vi "ReadBuffer.vi"(8 "error in (no error)":errorcluster, 11 "Arduino in":refnum<class "Arduino.lvclass">) -> (0 "error out":errorcluster, 2 "New Data Found":bool, 3 "Arduino out":refnum<class "Arduino.lvclass">)   [LabVIEW 2014, in "Arduino.lvclass"]
uses:
  Arduino.lvclass
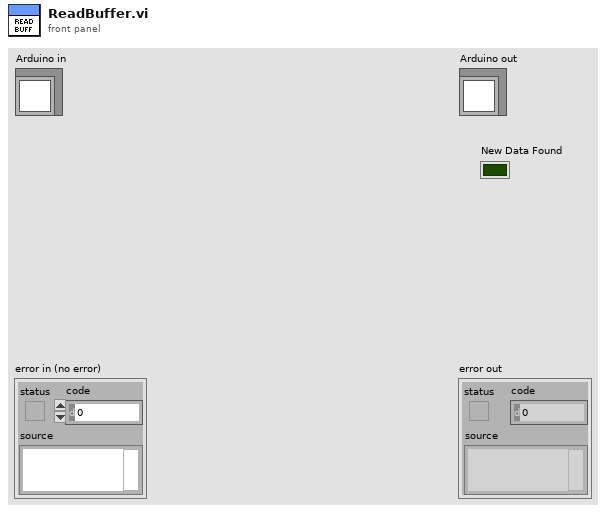
[diagram p1: front panel]
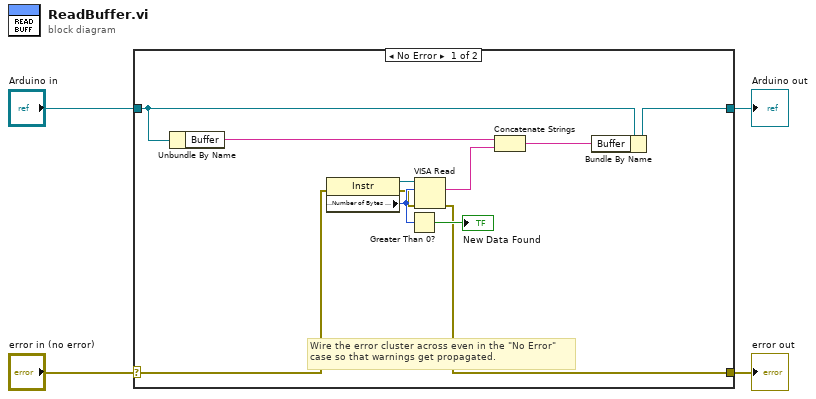
[diagram p0: block diagram]
diagram:
  n1 = case shown="No Error" "error in (no error)" {
    selector: "error in (no error)" -> [w10 w17]
    tunnel: [w11 w17] -> w3
    tunnel: [w5 w16] -> w1
    tunnel: "Arduino in" -> [w6 w16]
    frame No Error {
      # "Wire the error cluster across even in the \"No Error\"\ncase so that warnings get propagated."
      n2 = Unbundle By Name(w6) -> ("Buffer"=w8:string)
      n3 = property class="Instr"(error in=w10) -> (reference out=w15:refnum<visa-resource-name>, error out=w12:errorcluster, "Serial Settings:Number of Bytes at Serial Port"=w14:u32)  [unwired: 1 in]
      n4 = Greater Than 0?(x=w14) -> (x > 0?=→"New Data Found":bool)
      n5 = VISA Read(VISA resource name=w15, byte count=w14, error in (no error)=w12) -> (read buffer=w9:string, error out=w11:errorcluster)  [unwired: 2 out]
      n6 = Concatenate Strings(w8, w9) -> (w7:string)
      n7 = Bundle By Name(cluster=w6, "Buffer"=w7) -> (w5:refnum<class "Arduino.lvclass">)
    }
    frame Error {
    }
  }
  "error out" <- w3
  "Arduino out" <- w1
